vi "inputView.vi"(10 "UserEvents in":refnum<class "UserEvents.lvclass">) -> ()   [LabVIEW 2013]
uses:
  <userlib>/Common/ILC/Configuration/InputChannels.ctl
  UserEvents/UserEvents.lvclass
  UserEvents/UserEvents.lvclass/UserEvents.ctl
  Typedefs/StateSelector.ctl
  <userlib>/Common/ILC/Configuration/ILCConfiguration.lvlib
panel:
  out "Input Channels":T1
  out "Ch5":i32
  out "Ch4":i32
  out "Ch3":i32
  out "Ch2":i32
  out "Ch1":i32
  out "SSI Encoder":i32
  out "Tachometer":u16
  out "2":bool
  out "1":bool
  # "ADCs"
  # "Limit Switches"
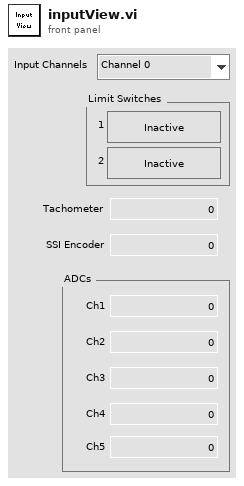
[diagram p1: front panel]
types:
  T1 = typedef "ILCCommon.lvlib/ILCConfiguration.lvlib/InputChannels.ctl" = enum16{"Channel 0", "3 Channels", "5 Channels"}
  T2 = typedef "PubDataEvents.ctl" = cluster{"State":refnum<user-event>, "ErrorCode":refnum<user-event>, "OutputData":refnum<user-event>, "InputData":refnum<user-event>, "ILCConfig":refnum<user-event>, "NeedUserOutputs":refnum<user-event>}
  T3 = cluster{"Event Registration Refnum":refnum<event-registration>, "Event Registration Refnum":refnum<event-registration>}
  T4 = typedef "StateSelector.ctl" = enum16{"DataOnDemandState", "DataStreamingState", "FaultState", "OffState", "StandbyState"}
  T5 = typedef "ILCCommon.lvlib/ILCTypedefs.lvlib/LimitSwitches.ctl" = cluster{"1":bool, "2":bool}
  T6 = typedef "ILCCommon.lvlib/ILCTypedefs.lvlib/ADCs.ctl" = cluster{"Ch1":i32, "Ch2":i32, "Ch3":i32, "Ch4":i32, "Ch5":i32}
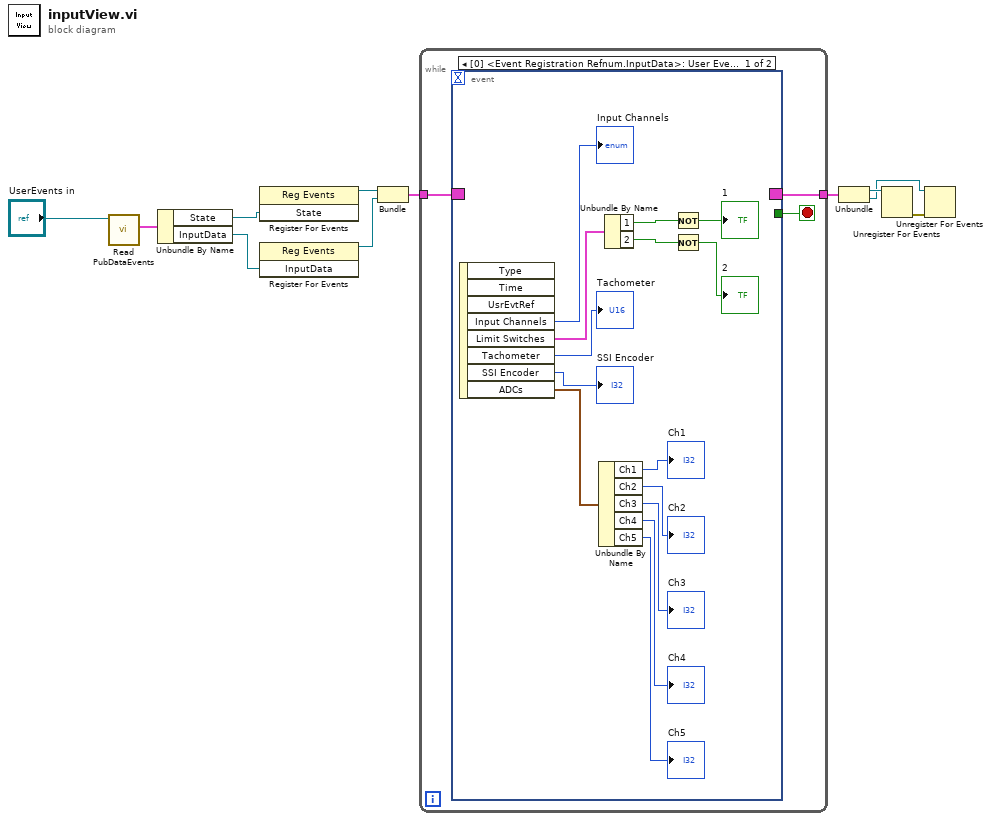
[diagram p0: block diagram]
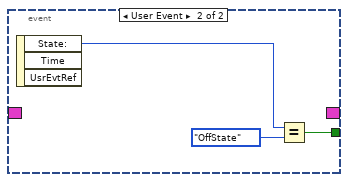
[diagram p2: hidden frame]
diagram:
  n1 = call "Read PubDataEvents.vi"("UserEvents in"="UserEvents in") -> ("PubDataEvents"=w11:T2)  [unwired: 9 in, 1 out]
  n2 = Unbundle By Name(w11) -> ("State"=w10:refnum<user-event>, "InputData"=w8:refnum<user-event>)
  n3 = register-events(w10) -> (reference out=w9:refnum<event-registration>)  [unwired: 2 in, 1 out]
  n4 = register-events(w8) -> (reference out=w7:refnum<event-registration>)  [unwired: 2 in, 1 out]
  n5 = Bundle("Event Registration Refnum"=w9, "Event Registration Refnum"=w7) -> (w5:T3)  [unwired: 1 in]
  n6 = while {
    tunnel: w5 -> [w14]
    tunnel: [w12] -> w4
    stop <- w13 stop-if-true
    n7 = event shown="[0] <Event Registration Refnum.InputData>: User Event" {
      selector: w14 -> [_ _]
      dyn-events: [_ _] -> w12
      timeout: _ -> [_ _]
      tunnel: [_ w30] -> w13
      event User Event {
        n8 = event-data() -> ("Input Channels"=→"Input Channels":T1, "Limit Switches"=w20:T5, "Tachometer"=→"Tachometer":u16, "SSI Encoder"=→"SSI Encoder":i32, "ADCs"=w17:T6)  [unwired: 1 in, 3 out]
        n9 = Unbundle By Name(w17) -> ("Ch1"=→"Ch1":i32, "Ch2"=→"Ch2":i32, "Ch3"=→"Ch3":i32, "Ch4"=→"Ch4":i32, "Ch5"=→"Ch5":i32)
        n10 = Unbundle By Name(w20) -> ("1"=w28:bool, "2"=w27:bool)
        n11 = Not(x=w28) -> (.not. x?=→"1":bool)
        n12 = Not(x=w27) -> (.not. x?=→"2":bool)
      }
      event User Event {
        n13 = event-data() -> ("State:"=w29:T4)  [unwired: 1 in, 2 out]
        n14 = Equal?(x=w29, y=StateSelector."OffState" ("State:")) -> (x = y?=w30:bool)
      }
    }
  }
  n15 = Unbundle(w4) -> ("Event Registration Refnum"=w3:refnum<event-registration>, "Event Registration Refnum"=w2:refnum<event-registration>)
  n16 = Unregister For Events(event registration refnum=w3) -> (error out=w1:errorcluster)  [unwired: 1 in]
  n17 = Unregister For Events(event registration refnum=w2, error in=w1) -> ()  [unwired: 1 out]
